vi "Trigger DAQ.vi"() -> ()   [LabVIEW 2020]
uses:
  SubVIs/MASTER.ctl
  SubVIs/Constants.ctl
  SubVIs/QBundle.ctl
  SubVIs/Queue.ctl
  SubVIs/Image data.ctl
  <vilib>/userdefined/High Color/IMAQdx.ctl
  <vilib>/vision/Image Controls.llb/IMAQ Image.ctl
  SubVIs/Image QBundle.ctl
panel:
  out "Image count":dbl
  in  "Digital output task":refnum<k21>
  in  "File type":string(combo)
  in  "Analog input task":refnum<k21>
  in  "Chart display tabs":T1(tab) caption="Display tabs"
  out "Analog Signals - Raw voltage":cluster{"Raw data[0]":dbl, "Raw data[1]":dbl}(graph)
  out "Analog Signals - Engineering units":cluster{"Engr data[0]":dbl, "Engr data[1]":dbl}(graph)
  in  "Scale (0) & Offset (1)":dbl[][](array[numeric])
  in  "AS #":string[](array[string])
  out "Channel Name":string[](array[string])
  out "Zero [V]":dbl[](array[numeric])
  out "Scale (0) & Offset (1)":dbl[][](array[numeric])
  in  "Enable":bool
  in  "Zero button":bool
  in  "Zero Signal [V]":dbl[](array[numeric])
  out "Analog Signals - Zero voltage":cluster{"Raw data[0]":dbl, "Raw data[1]":dbl}(graph)
  in  "Time":u16(ring) items=["Absolute time", "Relative time"]
  out "Timestamp [s]":dbl
  in  "Record data":bool
  in  "Sampling frequency [Hz]":dbl format="%#_10g"
  in  "Stop":bool
  in  "File Folder":path
  # "Records analog data at specified rate. Writes raw voltage data to CSV file."
  # "Recording parameters- do not change while program is running"
  # "Recording indicators"
  # "Controls"
  # "Instructions: \n1. Click file icon to select file folder\n2. Select file type. Default is a CSV file. \n3. Set the sample frequency for data acquisition. Default is 1 Hz. \n4. Select analog input task\n5. Select digital output task\n6. Select type of timestamp\n7. Run program with white arrow in tool bar\n8. Use controls to record data adn trigger cameras\n9. Zero raw data on 'ZERO' tab. Zeroed data is recorded as raw data when 'Enable' button is on. \n10. Scale chart to engineering units on 'ENGR' tab\n11. Record AS number of sensors on 'Channel Info' tab\n12. Stop program with 'STOP' button"
  # "Note: If editing number of channels in DAQmx task, seek help from Instrumentation team. Chart cluster size & historical data constant must be adjusted in back panel."
  # "Scale [Unit/V] & Offset [Unit]"
  # "Channel Information"
  # "Offset [Unit]"
  # "Scale [Unit/V]"
  # "Zeroed data is recorded as raw data when Enable button is on."
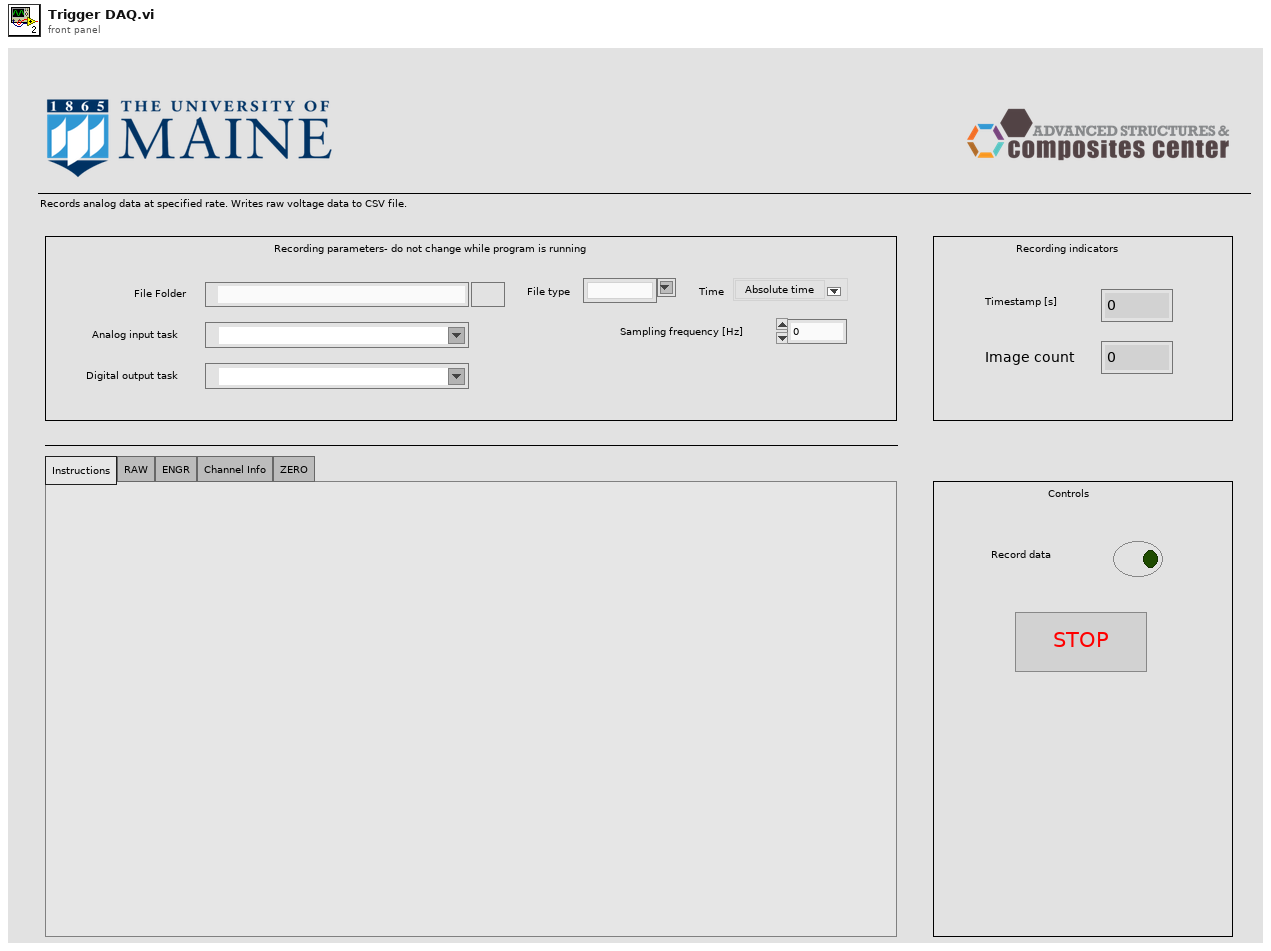
[diagram p1: front panel]
types:
  T1 = enum32{"Instructions", "RAW", "ENGR", "Channel Info", "ZERO"}
  T2 = typedef "MASTER.ctl" = cluster{"Constants":T3, "Queue Bundle":T4, "Queue":T5, "Image data":T6, "Image QBundle ":T9}
  T3 = typedef "Constants.ctl" = cluster{"Time":u16, "Samp. freq. [Hz]":dbl, "Samp. per chan.":i32, "Avg. div.":i32, "File path":path, "AI":refnum<k21>, "Loop 1 [Hz]":dbl, "Loop 2 [Hz]":dbl, "Loop 3 [Hz]":dbl, "Loop 1 [ms]":dbl, "Loop 2 [ms]":dbl, "Loop 3 [ms]":dbl, "Q1 buffer size":i32, "Q2 buffer size":i32, "File type":string, "Loop 4 [Hz]":dbl, "Loop 4 [ms]":dbl, "Channel Name":string[], "AS #":string[], "DO":refnum<k21>}
  T4 = typedef "QBundle.ctl" = cluster{"queue 1":refnum<queue>, "error 1":errorcluster, "queue 2":refnum<queue>, "error 2":errorcluster}
  T5 = typedef "Queue.ctl" = cluster{"Enable zero":bool, "Engr data [Unit]":dbl[], "Zero button":bool, "Zero [V]":dbl[], "Timestamp [s]":dbl, "Write sample":bool, "Record control":bool, "Stop":bool, "error":errorcluster, "Raw data [V]\n(all samples)":dbl[][], "Raw data [V]":dbl[], "Loop count":i64, "Initial time [s]":dbl, "Scale (0) & Offset (1)":dbl[][], "Image count":dbl}
  T6 = typedef "Image data.ctl" = cluster{"Camera 1":T7, "Camera 2":T7, "C1 Image out ":T8, "C2 Image out":T8, "C1 Model Name":string, "C1 Model Name 2":string, "Exposure time [us]":dbl, "Color Palette":u16, "C1 Buffer array":T8[], "Ready":bool, "C2 Buffer array":T8[]}
  T7 = typedef "IMAQdx.ctl" = refnum<k21>
  T8 = typedef "IMAQ Image.ctl" = refnum<image>
  T9 = typedef "Image QBundle.ctl" = cluster{"queue 1":refnum<queue>, "error 1":errorcluster, "queue 2":refnum<queue>, "error 2":errorcluster}
  T10 = cluster{"Engr data[0]":dbl, "Engr data[1]":dbl}[]
  T11 = cluster{"Engr data [Unit][0]":dbl, "Engr data [Unit][1]":dbl}
  T12 = cluster{"Raw data [V][0]":dbl, "Raw data [V][1]":dbl}
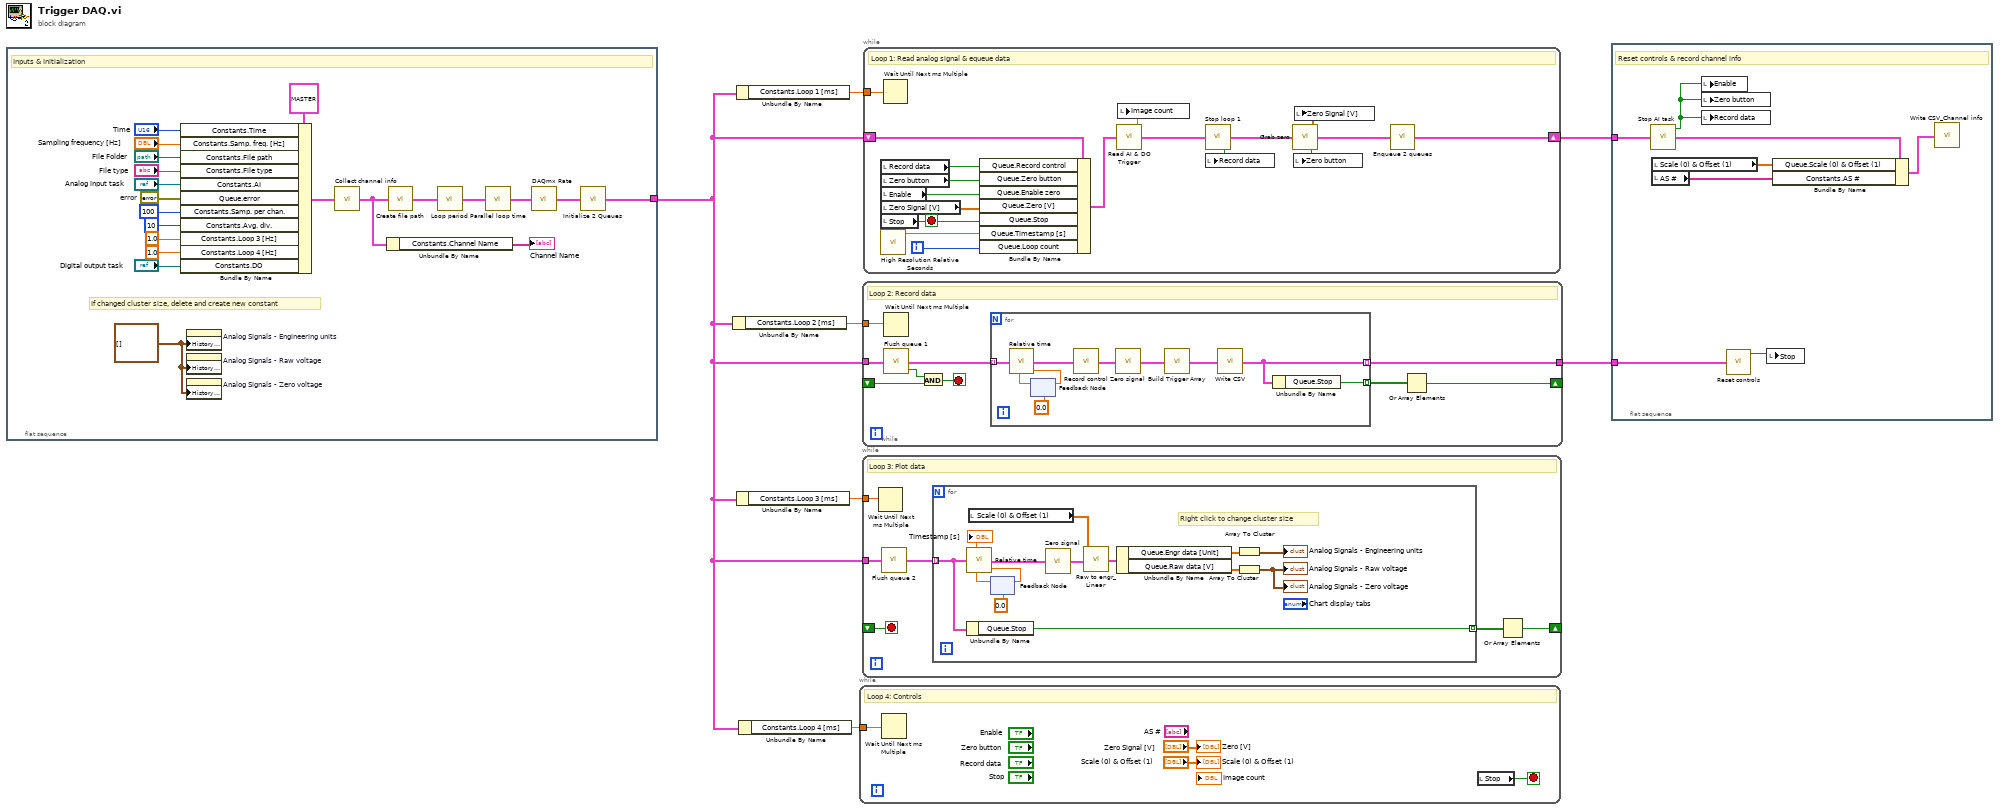
[diagram p0: block diagram]
diagram:
  n1 = flat-sequence {
    tunnel: [w28] -> w6
    frame #0 {
      w16 = errorcluster {"status"=FALSE, "code"=0, "source"=""}  # error
      w27 = T10 [] ("History Data")
      # "If changed cluster size, delete and create new constant"
      # "Inputs & Initialization"
      n2 = Bundle By Name(cluster=T2 {"Constants"={"Time"=0, "Samp. freq. [Hz]"=0.0, "Samp. per chan."=0, "Avg. div."=0, "File path"=path "", "AI"="", "Loop 1 [Hz]"=0.0, "Loop 2 [Hz]"=0.0, "Loop 3 [Hz]"=0.0, "Loop 1 [ms]"=0.0, "Loop 2 [ms]"=0.0, "Loop 3 [ms]"=0.0, "Q1 buffer size"=0, "Q2 buffer size"=0, "File type"="", "Loop 4 [Hz]"=0.0, "Loop 4 [ms]"=0.0, "Channel Name"=[], "AS #"=[], "DO"=""}, "Queue Bundle"={"queue 1"=refnum, "error 1"={"status"=FALSE, "code"=0, "source"=""}, "queue 2"=refnum, "error 2"={"status"=FALSE, "code"=0, "source"=""}}, "Queue"={"Enable zero"=FALSE, "Engr data [Unit]"=[], "Zero button"=FALSE, "Zero [V]"=[], "Timestamp [s]"=0.0, "Write sample"=FALSE, "Record control"=FALSE, "Stop"=FALSE, "error"={"status"=FALSE, "code"=0, "source"=""}, "Raw data [V]\n(all samples)"=[], "Raw data [V]"=[], "Loop count"=0, "Initial time [s]"=0.0, "Scale (0) & Offset (1)"=[], "Image count"=0.0}, "Image data"={"Camera 1"="", "Camera 2"="", "C1 Image out "=refnum, "C2 Image out"=refnum, "C1 Model Name"="", "C1 Model Name 2"="", "Exposure time [us]"=0.0, "Color Palette"=0, "C1 Buffer array"=[], "Ready"=FALSE, "C2 Buffer array"=[]}, "Image QBundle "={"queue 1"=refnum, "error 1"={"status"=FALSE, "code"=0, "source"=""}, "queue 2"=refnum, "error 2"={"status"=FALSE, "code"=0, "source"=""}}} ("Variables"), "Constants.Time"="Time", "Constants.Samp. freq. [Hz]"="Sampling frequency [Hz]", "Constants.File path"="File Folder", "Constants.File type"="File type", "Constants.AI"="Analog input task", "Queue.error"=w16, "Constants.Samp. per chan."=100 ("Samp. per chan."), "Constants.Avg. div."=10 ("Avg. div."), "Constants.Loop 3 [Hz]"=1.0 ("Loop 1 [ms]"), "Constants.Loop 4 [Hz]"=1.0 ("Loop 4 [Hz]"), "Constants.DO"="Digital output task") -> (w11:T2)
      n3 = property on="Analog Signals - Engineering units" class="WFChart (strict)"("History Data"=w27) -> ()  [unwired: 2 in, 2 out]
      n4 = property on="Analog Signals - Raw voltage" class="WFChart (strict)"("History Data"=w27) -> ()  [unwired: 2 in, 2 out]
      n5 = property on="Analog Signals - Zero voltage" class="WFChart (strict)"("History Data"=w27) -> ()  [unwired: 2 in, 2 out]
      n6 = call "Collect channel info.vi"("MASTER in"=w11) -> ("MASTER out"=w9:T2)  [unwired: 4 in]
      n7 = Unbundle By Name(w9) -> ("Constants.Channel Name"=→"Channel Name":string[])
      n8 = call "Create file path.vi"("MASTER in"=w9) -> ("MASTER out"=w25:T2)  [unwired: 4 in]
      n9 = call "Loop period.vi"("MASTER in"=w25) -> ("MASTER out"=w22:T2)  [unwired: 4 in]
      n10 = call "Parallel loop time.vi"("MASTER in"=w22) -> ("MASTER out"=w26:T2)  [unwired: 4 in]
      n11 = call "DAQmx Rate.vi"("MASTER in"=w26) -> ("MASTER out"=w10:T2)  [unwired: 4 in]
      n12 = call "Initialize 2 Queues.vi"("MASTER in"=w10) -> ("MASTER out"=w28:T2)  [unwired: 4 in]
    }
  }
  n13 = Unbundle By Name(w6) -> ("Constants.Loop 2 [ms]"=w3:dbl)
  n14 = Unbundle By Name(w6) -> ("Constants.Loop 1 [ms]"=w4:dbl)
  n15 = Unbundle By Name(w6) -> ("Constants.Loop 3 [ms]"=w2:dbl)
  n16 = Unbundle By Name(w6) -> ("Constants.Loop 4 [ms]"=w1:dbl)
  n17 = while {
    tunnel: w1 -> [w32]
    stop <- w29 stop-if-true
    # "Loop 4: Controls"
    n18 = Wait Until Next ms Multiple(millisecond multiple=w32) -> ()  [unwired: 1 out]
    n19 = local read "Stop"() -> (w29:bool)
    "Scale (0) & Offset (1)" <- "Scale (0) & Offset (1)"
    "Zero [V]" <- "Zero Signal [V]"
  }
  n20 = while {
    tunnel: w3 -> [w41]
    shift-right: [w39] -> _
    shift-left: _ -> [w37]
    tunnel: w6 -> [w36]
    tunnel: [w33] -> w5
    stop <- w38 stop-if-true
    # "Loop 2: Record data"
    n21 = Wait Until Next ms Multiple(millisecond multiple=w41) -> ()  [unwired: 1 out]
    n22 = call "Flush queue 1.vi"("MASTER in"=w36) -> ("MASTER array"=w34:T2[], "Zero elements in queue"=w35:bool)  [unwired: 5 in]
    n23 = And(x=w35, y=w37) -> (x .and. y?=w38:bool)
    n24 = for {
      tunnel: [w51] -> w40 mode=indexing
      tunnel: w34 -> [w48] mode=indexing
      tunnel: [w49] -> w33 mode=indexing
      n25 = feedback #1(0.0 ("Initial time out")) -> (w44:dbl)
      n26 = call "Relative time.vi"("MASTER in"=w48, "Initial time in"=w44) -> ("Initial time out"=w45:dbl, "MASTER out"=w47:T2)  [unwired: 3 in, 1 out]
      n27 = feedback-in #1(w45) -> ()
      n28 = call "Record control.vi"("MASTER in"=w47) -> ("MASTER out"=w50:T2)  [unwired: 4 in]
      n29 = call "Zero signal.vi"("MASTER in"=w50) -> ("MASTER out"=w43:T2)  [unwired: 6 in]
      n30 = call "Build Trigger Array.vi"("MASTER in"=w43) -> ("MASTER out"=w42:T2)  [unwired: 4 in]
      n31 = call "Write CSV.vi"("MASTER in"=w42) -> ("MASTER out"=w49:T2)  [unwired: 4 in]
      n32 = Unbundle By Name(w49) -> ("Queue.Stop"=w51:bool)
    }
    n33 = Or Array Elements(Boolean array=w40) -> (logical OR=w39:bool)
  }
  n34 = while {
    tunnel: w2 -> [w57]
    shift-right: [w55] -> _
    shift-left: _ -> [w54]
    tunnel: w6 -> [w52]
    stop <- w54 stop-if-true
    # "Loop 3: Plot data"
    n35 = Wait Until Next ms Multiple(millisecond multiple=w57) -> ()  [unwired: 1 out]
    n36 = call "Flush queue 2.vi"("MASTER in"=w52) -> ("MASTER array"=w53:T2[])  [unwired: 3 in, 1 out]
    n37 = for {
      tunnel: w53 -> [w68] mode=indexing
      tunnel: [w71] -> w56 mode=indexing
      # "Right click to change cluster size"
      n38 = Unbundle By Name(w68) -> ("Queue.Stop"=w71:bool)
      n39 = local read "Scale (0) & Offset (1)"() -> (w62:dbl[][])
      n40 = feedback #2(0.0 ("Initial time out")) -> (w65:dbl)
      n41 = call "Relative time.vi"("MASTER in"=w68, "Initial time in"=w65) -> ("Timestamp"=→"Timestamp [s]":dbl, "Initial time out"=w67:dbl, "MASTER out"=w64:T2)  [unwired: 3 in]
      n42 = feedback-in #2(w67) -> ()
      n43 = call "Zero signal.vi"("MASTER in"=w64) -> ("MASTER out"=w63:T2)  [unwired: 6 in]
      n44 = call "Raw to engr_Linear.vi"("MASTER in"=w63, "Slope (0) & Offset (1)"=w62) -> ("MASTER out"=w61:T2)  [unwired: 3 in]
      n45 = Unbundle By Name(w61) -> ("Queue.Engr data [Unit]"=w59:dbl[], "Queue.Raw data [V]"=w60:dbl[])
      n46 = Array To Cluster(array=w59) -> (cluster=→"Analog Signals - Engineering units":T11)
      n47 = Array To Cluster(array=w60) -> (cluster=→"Analog Signals - Raw voltage" →"Analog Signals - Zero voltage":T12)
    }
    n48 = Or Array Elements(Boolean array=w56) -> (logical OR=w55:bool)
  }
  n49 = while {
    tunnel: w4 -> [w89]
    shift-right: [w78] -> w7
    shift-left: w6 -> [w75]
    i -> [w80]
    stop <- w81 stop-if-true
    # "Loop 1: Read analog signal & equeue data"
    n50 = local read "Record data"() -> (w83:bool)
    n51 = local read "Zero button"() -> (w86:bool)
    n52 = local read "Enable"() -> (w85:bool)
    n53 = local read "Zero Signal [V]"() -> (w84:dbl[])
    n54 = local read "Stop"() -> (w81:bool)
    n55 = call <vilib>:"High Resolution Relative Seconds.vi"() -> ("relative seconds"=w88:dbl)
    n56 = Wait Until Next ms Multiple(millisecond multiple=w89) -> ()  [unwired: 1 out]
    n57 = Bundle By Name(cluster=w75, "Queue.Record control"=w83, "Queue.Zero button"=w86, "Queue.Enable zero"=w85, "Queue.Zero [V]"=w84, "Queue.Stop"=w81, "Queue.Timestamp [s]"=w88, "Queue.Loop count"=w80) -> (w74:T2)
    n58 = call "Read AI & DO Trigger.vi"("MASTER in"=w74) -> ("MASTER out"=w73:T2, "Image count"=w72:dbl)  [unwired: 3 in]
    n59 = local write "Image count"(w72) -> ()
    n60 = call "Stop loop 1.vi"("MASTER in"=w73) -> ("Record out"=w77:bool, "MASTER out"=w76:T2)  [unwired: 3 in]
    n61 = local write "Record data"(w77) -> ()
    n62 = call "Grab zero.vi"("MASTER in"=w76) -> ("Zero button"=w82:bool, "MASTER out"=w79:T2, "Zeros"=w87:dbl[])  [unwired: 2 in]
    n63 = local write "Zero button"(w82) -> ()
    n64 = local write "Zero Signal [V]"(w87) -> ()
    n65 = call "Enqueue 2 queues.vi"("MASTER in"=w79) -> ("MASTER out"=w78:T2)  [unwired: 4 in]
  }
  n66 = flat-sequence {
    tunnel: w7 -> [w97]
    tunnel: w5 -> [w91]
    frame #0 {
      # "Reset controls & record channel info"
      n67 = call "Stop AI task.vi"("MASTER in"=w97) -> ("MASTER out"=w94:T2, "Reset controls (F)"=w96:bool)  [unwired: 3 in]
      n68 = local read "Scale (0) & Offset (1)"() -> (w95:dbl[][])
      n69 = local read "AS #"() -> (w93:string[])
      n70 = local write "Enable"(w96) -> ()
      n71 = local write "Zero button"(w96) -> ()
      n72 = local write "Record data"(w96) -> ()
      n73 = call "Reset controls.vi"("MASTER Array in"=w91) -> ("Reset controls (F)"=w90:bool)  [unwired: 3 in, 1 out]
      n74 = local write "Stop"(w90) -> ()
      n75 = Bundle By Name(cluster=w94, "Queue.Scale (0) & Offset (1)"=w95, "Constants.AS #"=w93) -> (w92:T2)
      n76 = call "Write CSV_Channel info.vi"("MASTER in"=w92) -> ()  [unwired: 4 in, 1 out]
    }
  }
